vi "Topo & GridSpectr_DriftCorrection_v3.vi"(6 "Internal use":string, 7 "Grid param":T2 {"height (m)" format="%#_6p"; "width (m)" format="%#_6p"; "center Y (m)" format="%#_6p"; "center X (m)" format="%#_6p"}, 8 "Error in (no error)":errorcluster, 9 "Points Y/Index Y":i32, 10 "Points X/Index X":i32, 11 "Method":enum16{"init", "run", "end"}(ring)=enum."end") -> (0 "Error out":errorcluster)   [LabVIEW 2014]
doc: "Example of a measurement VI to be used in the \"Experiments on a Grid\" tool as external VI.\n\nThis example measure the topography and spectroscopy data. The spectroscopy measurements are taken on a subgrid. The data are saved to a sxm and a binary file.\n\n- Nanonis Programming Interface -"
uses:
  <userlib>/Nanonis Prog Interface V5/Nanonis Prog Interface.lvlib
panel:
  in  "Drift Correction 2":T1
  out "Numeric":i32
  out "X drift":i32
  out "Y drift":i32
  out "Queue Steps":i32
  in  "StepsBack":i32
  in  "Channel index (0-23)":u8=14
  in  "File name":string
  in  "STS Current":dbl format="%#_6p"
  in  "Imaging Current":dbl format="%#_6p"
  in  "zdrift \nDuration (s)":dbl
  in  "Correct z drift":bool
  out "Status":string="init"
  in  "Drift correction Pixels":i32=128 caption="Pixels for drift correction"
  out "Y Offset":dbl
  out "X Offset":dbl
  out "Points taken":dbl=1.0
  in  "Drift Correction":i32=128
  in  "Y subgrid spacing":u16=1
  in  "X subgrid spacing":u16=1
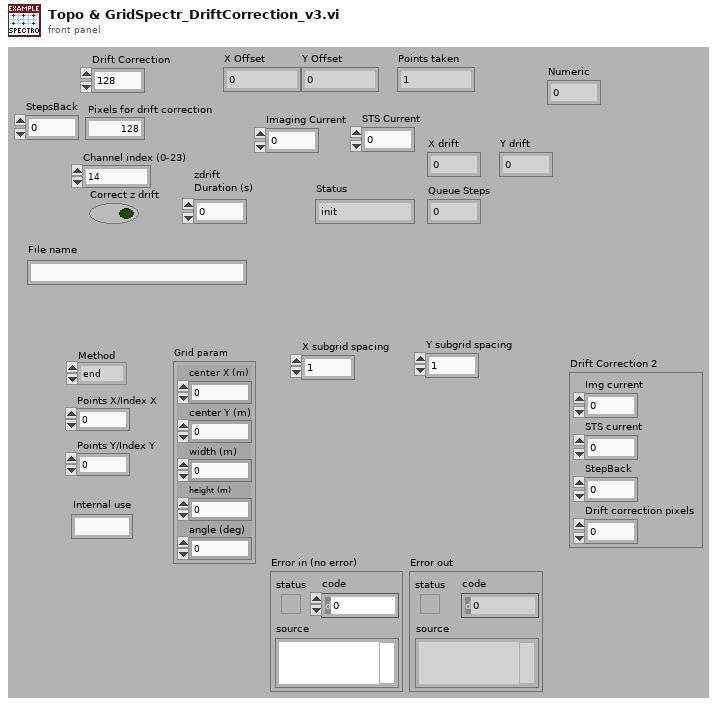
[diagram p1: front panel]
types:
  T1 = cluster{"Img current":dbl, "STS current":dbl, "StepBack":dbl, "Drift correction pixels":dbl}
  T2 = cluster{"center X (m)":sgl, "center Y (m)":sgl, "width (m)":sgl, "height (m)":sgl, "angle (deg)":sgl}
  T3 = cluster{"center X":sgl, "center Y":sgl, "angle":sgl, "width":sgl, "height":sgl, "# pixels":i32, "# lines":i32}
  T4 = cluster{"Name":string, "Calibration":sgl, "Offset":sgl, "Channel index":i32}[]
  T5 = cluster{"up/down":bool, "time/line":sgl, "start time":timestamp, "end time":timestamp}
  T6 = cluster{"Z averaging time (s)":sgl, "Z offset (m)":sgl, "Initial settling time (s)":sgl}
  T7 = cluster{"Max. slew rate (V/s)":sgl, "Settling time (s)":sgl, "Integration time (s)":sgl}
  T8 = cluster{"End settling time (s)":sgl, "Z control time (s)":sgl}
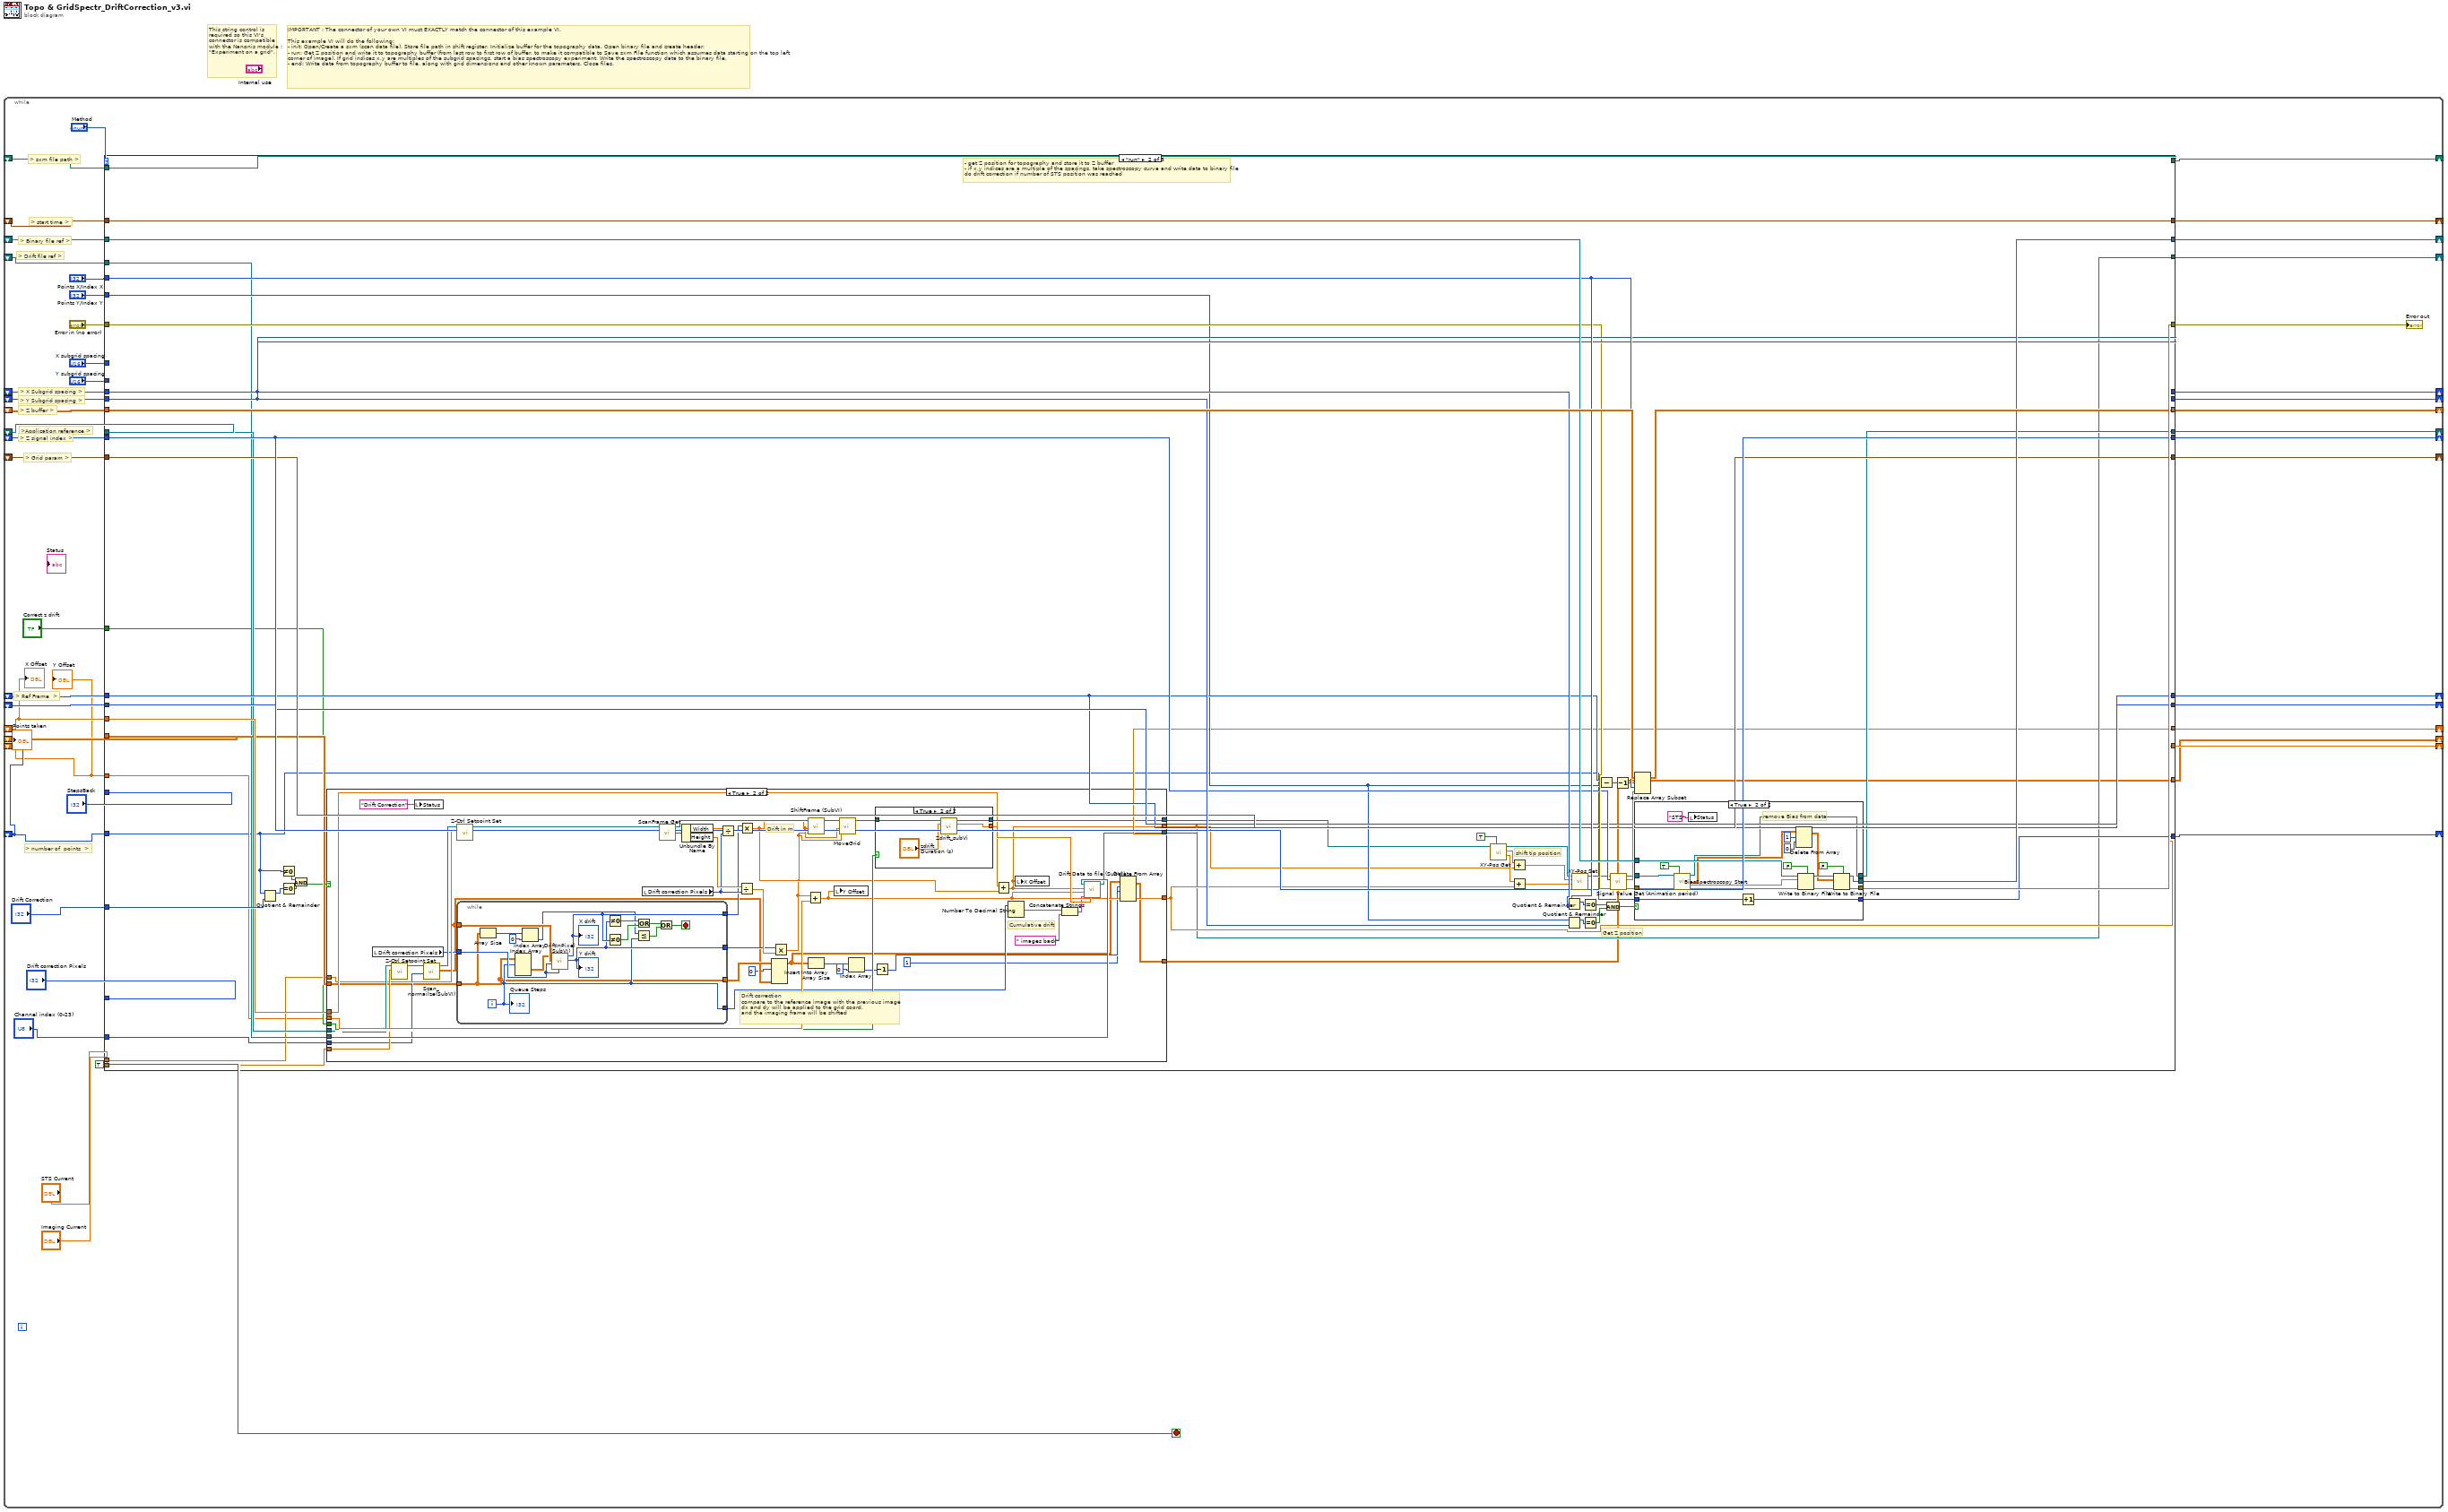
[diagram p0: block diagram]
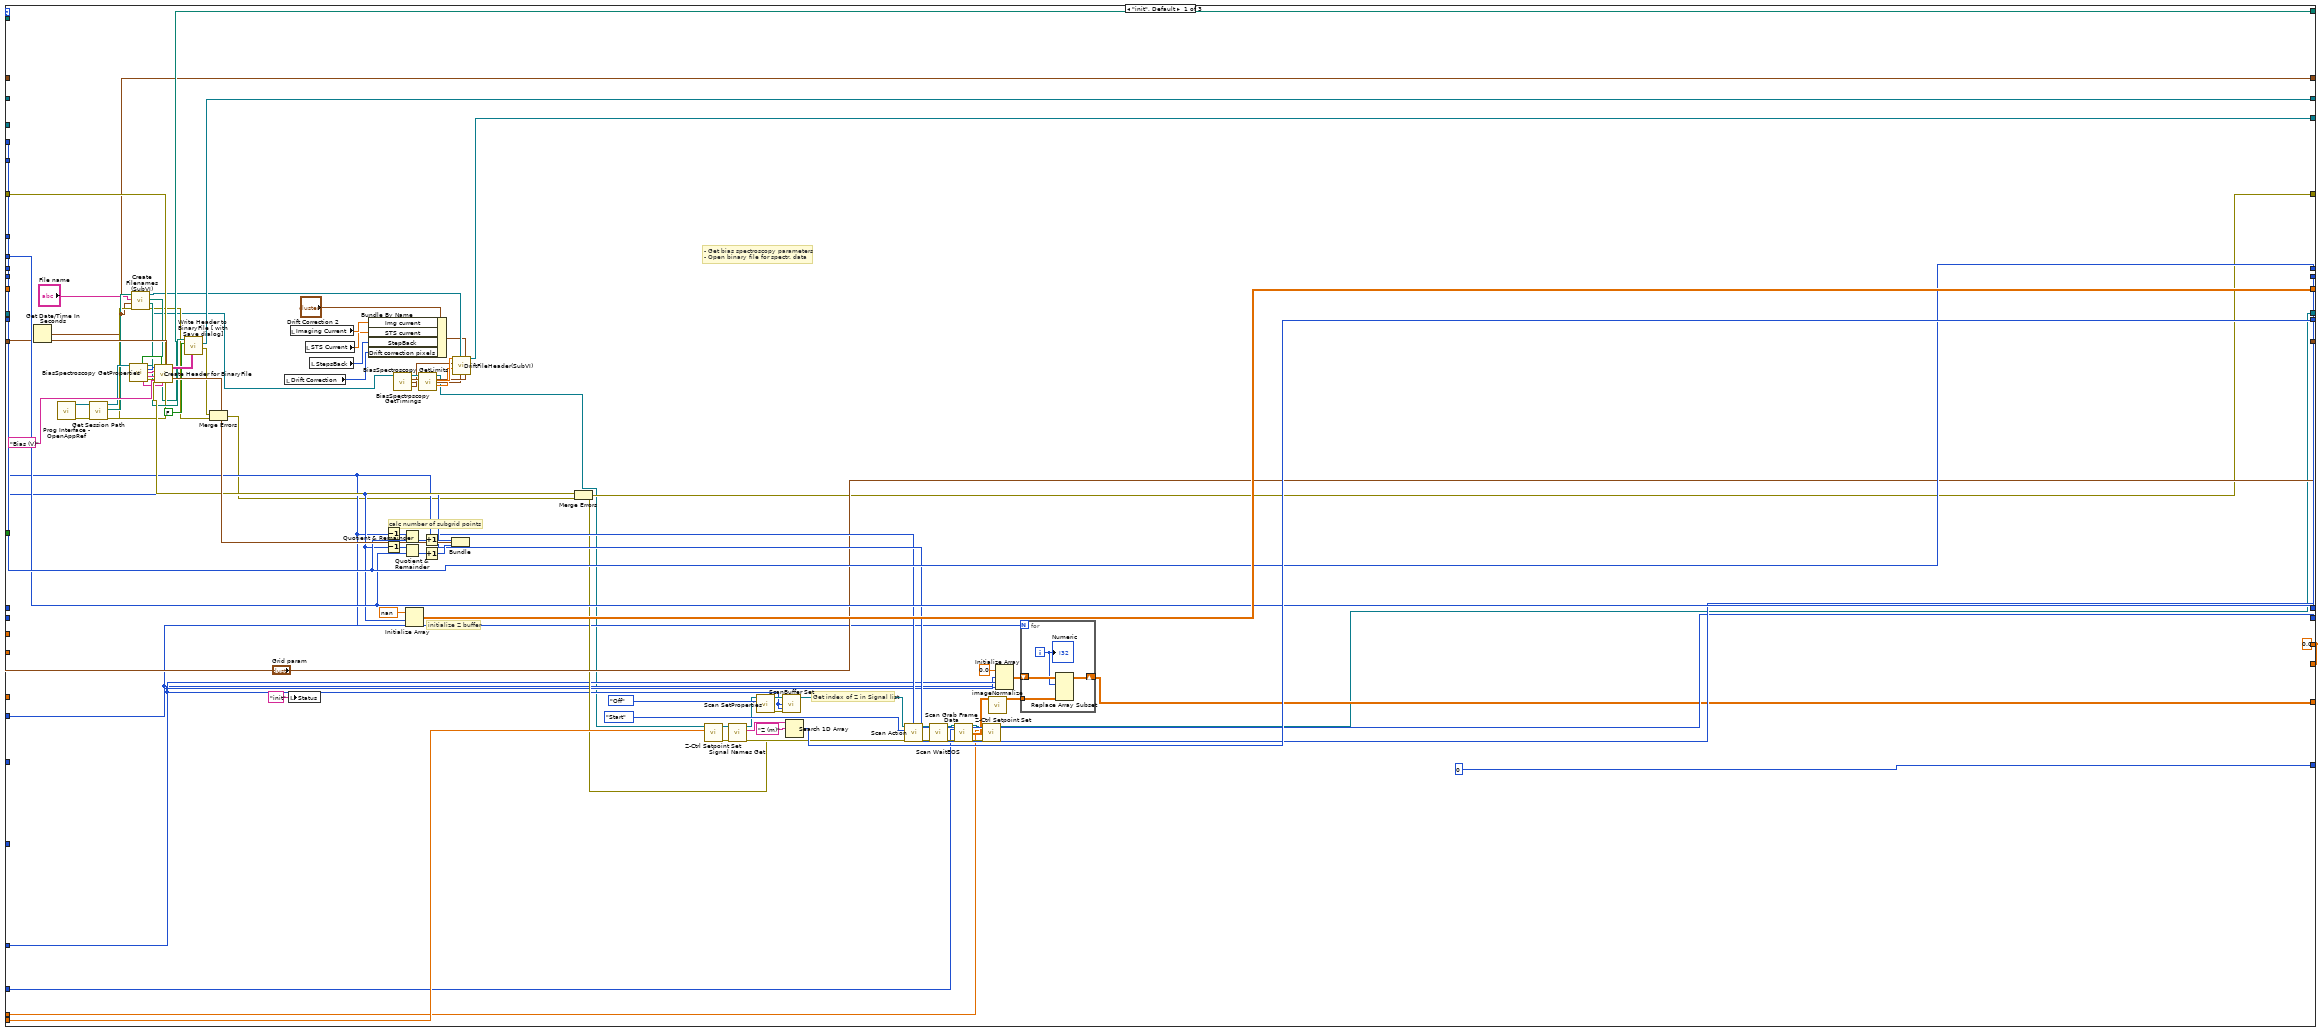
[diagram p2: hidden frame]
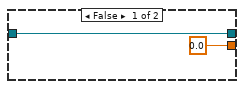
[diagram p4: hidden frame]
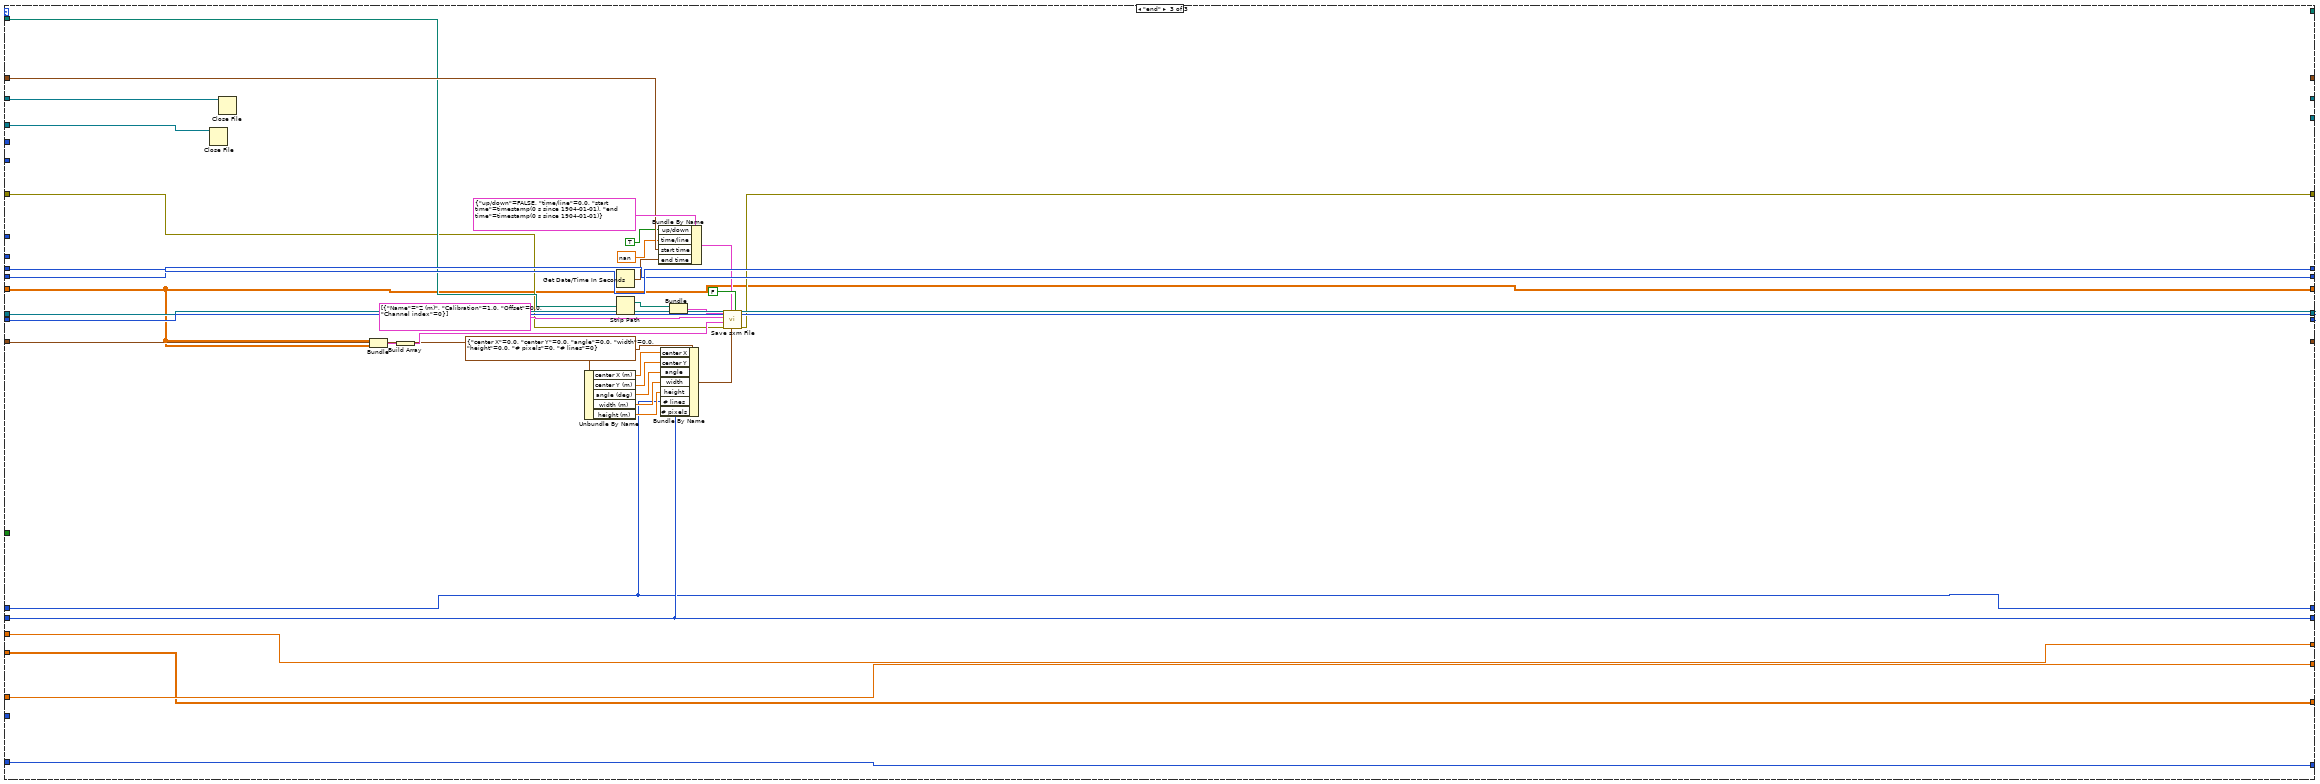
[diagram p6: hidden frame]
diagram:
  # "This string control is required so this VI's connector is compatible with the Nanonis module : \"Experiment on a grid\"."
  # "IMPORTANT : The connector of your own VI must EXACTLY match the connector of this example VI.\n\nThis example VI will do the following:\n- init: Open/Create a sxm (scan data file). Store file path in shift register. Initialize buffer for the topography data. Open binary file and create header.\n- run: Get Z position and write it to topography buffer (from last row to first row of buffer, to make it compatible to Save sxm File function which assumes data starting on the top left corner of image). If grid indices x,y are multiples of the subgrid spacings, start a bias spectroscopy experiment. Write the spectroscopy data to the binary file.\n- end: Write data from topography buffer to file, along with grid dimensions and other known parameters. Close files."
  n1 = while {
    shift-right: [w22] -> _
    shift-left: _ -> [w45]
    shift-right: [w40] -> _
    shift-left: _ -> [w39]
    shift-right: [w37] -> _
    shift-left: _ -> [w38]
    shift-right: [w36] -> _
    shift-left: _ -> [w35]
    shift-right: [w29] -> _
    shift-left: _ -> [w31]
    shift-right: [w30] -> _
    shift-left: _ -> [w32]
    shift-right: [w28] -> _
    shift-left: _ -> [w27]
    shift-right: [w26] -> _
    shift-left: _ -> [w25]
    shift-right: [w24] -> _
    shift-left: _ -> [w23]
    shift-right: [w21] -> _
    shift-left: _ -> [w20]
    shift-right: [w19] -> _
    shift-left: _ -> [w18]
    shift-right: [w17] -> _
    shift-left: _ -> [w10]
    shift-right: [w16] -> _
    shift-left: _ -> [w9]
    shift-right: [w15] -> _
    shift-left: _ -> [w12]
    shift-right: [w14] -> _
    shift-left: _ -> [w11]
    shift-right: [w7] -> _
    shift-left: _ -> [w6]
    stop <- TRUE stop-if-true
    # "> Drift file ref >"
    # "> number of  points  >"
    # "> Ref Frame  >"
    # "> Grid param >"
    # "> start time >"
    # ">Application reference >"
    # "> Y Subgrid spacing >"
    # "> X Subgrid spacing >"
    # "> Z signal index >"
    # "> Binary file ref >"
    # "> Z buffer >"
    # "> sxm file path >"
    n2 = case shown="\"run\"" "Method" {
      tunnel: [w77 w192 _] -> w22
      tunnel: w45 -> [_ w192 w315]
      tunnel: "Error in (no error)" -> [w79 w178 w308]
      tunnel: [w88 w191 w307] -> w43
      tunnel: "Points X/Index X" -> [w109 w186 _]
      tunnel: "Points Y/Index Y" -> [w110 w170 _]
      tunnel: [w133 w189 w296] -> w40
      tunnel: w39 -> [_ w190 w296]
      tunnel: w38 -> [_ w188 w324]
      tunnel: [w125 w187 _] -> w37
      tunnel: [w123 w176 w325] -> w36
      tunnel: w35 -> [_ w176 w325]
      tunnel: "X subgrid spacing" -> [w122 _ _]
      tunnel: "Y subgrid spacing" -> [w121 _ _]
      tunnel: w32 -> [_ w180 w323]
      tunnel: w31 -> [_ w179 w322]
      tunnel: [w122 w180 w323] -> w30
      tunnel: [w121 w179 w322] -> w29
      tunnel: [w50 w162 w321] -> w28
      tunnel: w27 -> [_ w161 w321]
      tunnel: ["Grid param" w173 _] -> w26
      tunnel: w25 -> [_ w173 w306]
      tunnel: [w76 w174 _] -> w24
      tunnel: w23 -> [_ w174 w316]
      tunnel: [w110 w171 w297] -> w21
      tunnel: w20 -> [_ w171 w297]
      tunnel: [w109 w172 w298] -> w19
      tunnel: w18 -> [_ w172 w298]
      tunnel: [w100 w146 w295] -> w17
      tunnel: [w100 w151 w293] -> w16
      tunnel: [w71 w143 w289] -> w15
      tunnel: [0 w167 w294] -> w14
      tunnel: w11 -> [_ w140 w294]
      tunnel: "Drift Correction" -> [_ w165 _]
      tunnel: w12 -> [_ w150 w289]
      tunnel: w10 -> [_ w163 w295]
      tunnel: w9 -> [_ w141 w293]
      tunnel: "Drift correction Pixels" -> [w70 _ _]
      tunnel: [w66 w148 _] -> w7
      tunnel: w6 -> [_ w149 w290]
      tunnel: "Correct z drift" -> [_ w147 _]
      tunnel: "Imaging Current" -> [w89 w145 _]
      tunnel: "STS Current" -> [w84 w144 _]
      tunnel: "Channel index (0-23)" -> [w74 w142 _]
      tunnel: "StepsBack" -> [w69 _ _]
      frame "init", Default {
        w100 = 0.0
        # "- Get bias spectroscopy parameters\n- Open binary file for spectr. data"
        # "initialize Z buffer"
        # "calc number of subgrid points"
        # "Get index of Z in Signal list"
        n3 = Get Date/Time In Seconds() -> (seconds since 1Jan1904=w76:timestamp)
        n4 = call <userlib>:"Prog Interface - OpenAppRef.vi"("Error in (no error)"=w79) -> ("Error out"=w81:errorcluster, "Application reference"=w83:refnum<vi>)  [unwired: 5 in]
        n5 = call <userlib>:"Get Session Path.vi"("error in (no error)"=w81, "Application ref in"=w83) -> ("error out"=w78:errorcluster, "Session path"=w80:path, "Application ref out"=w82:refnum<vi>)  [unwired: 7 in]
        n6 = call <userlib>:"BiasSpectroscopy GetProperties.vi"("Application ref in"=w82) -> ("Backward sweep"=w129:bool, "Application ref out"=w49:refnum<vi>, "Number of points"=w112:i32, "Channels"=w111:string[], "Parameters"=w127:string[], "Fixed parameters"=w114:string[], "Error out"=w126:errorcluster)  [unwired: 6 in, 2 out]
        n7 = call "Create Filenames (SubVI).vi"("error in (no error)"=w78, "seconds since 1Jan1904"=w76, "File name"="File name", "Session path"=w80) -> ("error out"=w51:errorcluster, "binFilePath"=w92:path, "topoFilePath"=w77:path, "Drift File out"=w67:refnum<file>)  [unwired: 4 in]
        n8 = local read "Drift Correction"() -> (w61:i32)
        n9 = local write "Status"("init" ("Status")) -> ()
        n10 = local read "Imaging Current"() -> (w63:dbl)
        n11 = local read "STS Current"() -> (w62:dbl)
        n12 = local read "StepsBack"() -> (w60:i32)
        n13 = Bundle By Name(cluster="Drift Correction 2", "Img current"=w63, "STS current"=w62, "StepBack"=w60, "Drift correction pixels"=w61) -> (w64:T1)
        n14 = Decrement(x=w109) -> (x-1=w120:i32)
        n15 = Decrement(x=w110) -> (x-1=w119:i32)
        n16 = call <userlib>:"BiasSpectroscopy GetTimings.vi"("Application ref in"=w49) -> ("Application ref out"=w59:refnum<vi>, "Initialization"=w56:T6, "Sweep Timing"=w54:T7, "End of Sweep"=w55:T8)  [unwired: 10 in, 1 out]
        n17 = Quotient & Remainder(x=w120, y=w122) -> (floor(x/y)=w118:i32)  [unwired: 1 out]
        n18 = Quotient & Remainder(x=w119, y=w121) -> (floor(x/y)=w117:i32)  [unwired: 1 out]
        n19 = Initialize Array(sgl nan ("element"), w110, w109) -> (w133:sgl[][])
        n20 = call <userlib>:"BiasSpectroscopy GetLimits.vi"("Application ref in"=w59) -> ("End value (V)"=w57:sgl, "Start value (V)"=w58:sgl, "Application ref out"=w48:refnum<vi>)  [unwired: 5 in, 1 out]
        n21 = Increment(x=w118) -> (x+1=w116:i32)
        n22 = Increment(x=w117) -> (x+1=w115:i32)
        n23 = Bundle(w116, w115) -> (w128:cluster{i32, i32})  [unwired: 1 in]
        n24 = call <userlib>:"Create Header for BinaryFile.vi"("Grid points"=w128, "Grid param"="Grid param", "Fixed parameters"=w114, "Backward sweep"=w129, "Sweep signal"="Bias (V)" ("Sweep Signal"), "Parameters"=w127, "Channels"=w111, "Points per sweep"=w112) -> ("Header (fixed attributes)"=w131:string[][])  [unwired: 3 in]
        n25 = call <userlib>:"Write Header to BinaryFile [ with Save dialog].vi"("Fixed Attributes"=w131, "Show Dialog? (T)"=FALSE, "Filename"=w92) -> ("Error out"=w52:errorcluster, "File ref"=w125:refnum<file>)  [unwired: 5 in, 2 out]
        n26 = Merge Errors(w52, w51) -> (w53:errorcluster)
        n27 = call "DriftFileHeader(SubVI).vi"("Initialization"=w56, "Drift Correction"=w64, "Sweep Timing"=w54, "Byte Stream File in"=w67, "End value (V)"=w57, "End of Sweep"=w55, "Start value (V)"=w58) -> ("Byte Stream File out"=w66:refnum<file>)  [unwired: 4 in]
        n28 = Merge Errors(w126, w53) -> (w88:errorcluster)
        n29 = call <userlib>:"Z-Ctrl Setpoint Set.vi"("error in (no error)"=w88, "Z Controller setpoint"=w89, "Application ref in"=w48) -> ("error out"=w87:errorcluster, "Application ref out"=w90:refnum<vi>)  [unwired: 7 in]
        n30 = call <userlib>:"Signal Names Get.vi"("error in (no error)"=w87, "Application ref in"=w90) -> ("error out"=w101:errorcluster, "Signals Names"=w113:string[], "Application ref out"=w96:refnum<vi>)  [unwired: 5 in]
        n31 = call <userlib>:"Scan SetProperties.vi"("Application ref in"=w96, "Continuous scan"=enum16{"No change", "On", "Off"}."Off") -> ("Application ref out"=w98:refnum<vi>, "Error out"=w97:errorcluster)  [unwired: 12 in]
        n32 = call <userlib>:"ScanBuffer Set.vi"("Application ref in"=w98, "Pixels"=w70, "Lines"=w70, "error in (no error)"=w97) -> ("Application ref out"=w95:refnum<vi>)  [unwired: 10 in, 1 out]
        n33 = Search 1D Array(1D array=w113, element="Z (m)") -> (index of element=w123:i32)  [unwired: 1 in]
        n34 = call <userlib>:"Scan Action.vi"("error in (no error)"=w101, "Scan action (Start)"=enum16{"Start", "Stop", "Pause", "Resume"}."Start", "Application ref in"=w95) -> ("error out"=w107:errorcluster, "Application ref out"=w106:refnum<vi>)  [unwired: 6 in]
        n35 = call <userlib>:"Scan WaitEOS.vi"("error in (no error)"=w107, "Application ref in"=w106) -> ("error out"=w104:errorcluster, "Application ref out"=w105:refnum<vi>)  [unwired: 5 in, 2 out]
        n36 = call <userlib>:"Scan Grab Frame Data.vi"("Application ref in"=w105, "Channel index (0-23)"=w74, "error in (no error)"=w104) -> ("Application ref out"=w86:refnum<vi>, "Scan frame data"=w91:sgl[][], "error out"=w85:errorcluster)  [unwired: 8 in, 2 out]
        n37 = call <userlib>:"Z-Ctrl Setpoint Set.vi"("error in (no error)"=w85, "Z Controller setpoint"=w84, "Application ref in"=w86) -> ("Application ref out"=w50:refnum<vi>)  [unwired: 7 in, 1 out]
        n38 = call "imageNormalize.vi"("Data"=w91) -> ("Array"=w68:dbl[][])  [unwired: 10 in]
        n39 = Initialize Array(0.0 ("element"), w69, w70, w70) -> (w72:dbl[][][])
        n40 = for {
          N: w69 -> [_]
          tunnel: w68 -> [w136]
          shift-right: [w135] -> w71
          shift-left: w72 -> [w137]
          i -> [w134]
          n41 = Replace Array Subset(array=w137, new element=w136, index (dim 0)=w134) -> (w135:dbl[][][])  [unwired: 2 in]
          "Numeric" <- w134
        }
      }
      frame "run" {
        # "shift tip position"
        # "Get Z position"
        # "- get Z position for topography and store it to Z buffer\n- if x,y indices are a multiple of the spacings, take spectroscopy curve and write data to binary file\ndo drift correction if number of STS position was reached"
        n42 = Quotient & Remainder(x=w140, y=w165) -> (x-y*floor(x/y)=w166:i32)  [unwired: 1 out]
        n43 = Not Equal To 0?(x=w140) -> (x != 0?=w138:bool)
        n44 = Equal To 0?(x=w166) -> (x = 0?=w164:bool)
        n45 = And(x=w138, y=w164) -> (x .and. y?=w139:bool)
        n46 = case shown="True" w139 {
          tunnel: w161 -> [w197 w228]
          tunnel: [w197 w234] -> w160
          tunnel: w150 -> [w194 w216]
          tunnel: [w196 w230] -> w146
          tunnel: [w195 w229] -> w151
          tunnel: w163 -> [w196 w232]
          tunnel: w141 -> [w195 w233]
          tunnel: [w194 w208] -> w143
          tunnel: w149 -> [w193 w237]
          tunnel: [w193 w236] -> w148
          tunnel: w147 -> [_ w231]
          tunnel: w145 -> [_ w227]
          tunnel: w144 -> [_ w225]
          tunnel: w142 -> [_ w220]
          frame False {
          }
          frame True {
            # "Cumulative drift"
            # "Drift in m"
            # "Drift correction \ncompare to the reference image with the previous image \ndx and dy will be applied to the grid coord, \nand the imaging frame will be shifted"
            n47 = local read "Drift correction Pixels"() -> (w219:i32)
            n48 = call <userlib>:"Z-Ctrl Setpoint Set.vi"("Z Controller setpoint"=w227, "Application ref in"=w228) -> ("Application ref out"=w224:refnum<vi>)  [unwired: 8 in, 1 out]
            n49 = local write "Status"("Drift Correction" ("Status")) -> ()
            n50 = call "Scan_normailze(SubVI).vi"("Channel index (0-23)"=w220, "Application in"=w224) -> ("Array"=w210:dbl[][], "Application out"=w226:refnum<vi>)  [unwired: 7 in, 1 out]
            n51 = call <userlib>:"Z-Ctrl Setpoint Set.vi"("Z Controller setpoint"=w225, "Application ref in"=w226) -> ("Application ref out"=w222:refnum<vi>)  [unwired: 8 in, 1 out]
            n52 = while {
              tunnel: w219 -> [w256]
              tunnel: w210 -> [w255]
              tunnel: w216 -> [w245]
              tunnel: [w254] -> w218
              tunnel: [w253] -> w217
              tunnel: [w249] -> w215
              tunnel: [w245] -> w211
              i -> [w249]
              stop <- w251 stop-if-true
              n53 = Array Size(array=w245) -> (size(s)=w248:i32[])
              n54 = Index Array(array=w245, index (dim 0)=w249) -> (element=w244:dbl[][])  [unwired: 2 in]
              n55 = Index Array(array=w248, index=0) -> (element=w246:i32)
              n56 = call "DriftInPixel (SubVI).vi"(6:w256, 9:w256, "New image"=w255, "Ref image"=w244) -> ("Y drift"=w253:i32, "X drift"=w254:i32)  [unwired: 5 in, 1 out]
              "Y drift" <- w253
              "X drift" <- w254
              n57 = Not Equal To 0?(x=w253) -> (x != 0?=w258:bool)
              n58 = Not Equal To 0?(x=w254) -> (x != 0?=w257:bool)
              n59 = Or(x=w258, y=w257) -> (x .or. y?=w252:bool)
              n60 = Less Or Equal?(x=w246, y=w249) -> (x <= y?=w250:bool)
              n61 = Or(x=w252, y=w250) -> (x .or. y?=w251:bool)
              "Queue Steps" <- w249
            }
            n62 = local read "Drift correction Pixels"() -> (w221:i32)
            n63 = call <userlib>:"ScanFrame Get.vi"("Application ref in"=w222) -> ("Application ref out"=w223:refnum<vi>, "Size (m)"=w242:cluster{"Width":sgl, "Height":sgl})  [unwired: 10 in, 3 out]
            n64 = Unbundle By Name(w242) -> ("Width"=w241:sgl, "Height"=w243:sgl)
            n65 = Divide(x=w241, y=w221) -> (x/y=w240:sgl)
            n66 = Divide(x=w243, y=w221) -> (x/y=w239:sgl)
            n67 = Multiply(x=w218, y=w240) -> (x*y=w199:sgl)
            n68 = Insert Into Array(array=w211, index (dim 0)=0 ("index (page)"), new element=w210) -> (w207:dbl[][][])  [unwired: 2 in]
            n69 = Multiply(x=w217, y=w239) -> (x*y=w198:sgl)
            n70 = Add(x=w198, y=w233) -> (x+y=w229:dbl)
            n71 = call "ShiftFrame (SubVI).vi"("Y shift"=w198, "X shift"=w199, "Application in"=w223) -> ("Application out"=w201:refnum<vi>)  [unwired: 8 in]
            n72 = Array Size(array=w207) -> (size(s)=w206:i32[])
            n73 = local write "Y Offset"(w229) -> ()
            n74 = call "MoveGrid.vi"("y"=w198, "x"=w199, "Application ref in"=w201) -> ("Application ref out"=w200:refnum<vi>)  [unwired: 7 in, 1 out]
            n75 = Index Array(array=w206, index=0) -> (element=w204:i32)
            n76 = Decrement(x=w204) -> (x-1=w203:i32)
            n77 = case shown="True" w231 {
              tunnel: [0.0 ("z drift") w264] -> w235
              tunnel: w200 -> [w259 w263]
              tunnel: [w259 w262] -> w234
              frame False {
              }
              frame True {
                n78 = call "Zdrift_subVi.vi"("Duration"="zdrift \nDuration (s)", "Application in"=w263) -> ("z drift"=w264:dbl, "Application out"=w262:refnum<vi>)  [unwired: 7 in, 1 out]
              }
            }
            n79 = Add(x=w232, y=w199) -> (x+y=w230:dbl)
            n80 = Number To Decimal String(number=w215) -> (decimal integer string=w214:string)  [unwired: 1 in]
            n81 = local write "X Offset"(w230) -> ()
            n82 = Concatenate Strings(w214, " images back" ("string")) -> (w213:string)
            n83 = call "Drift Data to file (SubVI).vi"("z drift"=w235, "Comment"=w213, "y Drift"=w229, "X drift"=w230, "Byte Stream File in"=w237) -> ("Byte Stream File out"=w236:refnum<file>)  [unwired: 6 in]
            n84 = Delete From Array(array=w207, length=1, index (dim 0)=w203) -> (array with subset deleted=w208:dbl[][][])  [unwired: 2 in, 1 out]
          }
        }
        n85 = call <userlib>:"XY-Pos Get.vi"("Wait for newest data (F=False)"=TRUE, "Application ref in"=w160) -> ("Y (m)"=w155:sgl, "X (m)"=w156:sgl, "Application ref out"=w157:refnum<vi>)  [unwired: 5 in, 1 out]
        n86 = Add(x=w156, y=w146) -> (x+y=w154:dbl)
        n87 = Add(x=w155, y=w151) -> (x+y=w153:dbl)
        n88 = Quotient & Remainder(x=w186, y=w180) -> (x-y*floor(x/y)=w185:i32)  [unwired: 1 out]
        n89 = Quotient & Remainder(x=w170, y=w179) -> (x-y*floor(x/y)=w184:i32)  [unwired: 1 out]
        n90 = call <userlib>:"XY-Pos Set.vi"("Y (m)"=w153, "X (m)"=w154, "Application ref in"=w157) -> ("Application ref out"=w158:refnum<vi>)  [unwired: 5 in, 1 out]
        n91 = Equal To 0?(x=w185) -> (x = 0?=w183:bool)
        n92 = Equal To 0?(x=w184) -> (x = 0?=w182:bool)
        n93 = Subtract(x=w171, y=w170) -> (x-y=w169:i32)
        n94 = And(x=w183, y=w182) -> (x .and. y?=w181:bool)
        n95 = call <userlib>:"Signal Value Get (Animation period).vi"("error in (no error)"=w178, "Signal index (0-47)"=w176, "Application ref in"=w158) -> ("error out"=w177:errorcluster, "Signal value"=w175:sgl, "Application ref out"=w159:refnum<vi>)  [unwired: 5 in]
        n96 = Decrement(x=w169) -> (x-1=w168:i32)
        n97 = Replace Array Subset(array=w190, new element=w175, index (row)=w168, index (col)=w186) -> (w189:sgl[][])
        n98 = case shown="True" w181 {
          tunnel: [w267 w272] -> w191
          tunnel: w188 -> [w268 w288]
          tunnel: [w268 w286] -> w187
          tunnel: w177 -> [w267 w285]
          tunnel: w159 -> [w266 w277]
          tunnel: [w266 w276] -> w162
          tunnel: [w265 w270] -> w167
          tunnel: w140 -> [w265 w271]
          frame False {
            # "Point indices aren't multiple of subgrid spacing\n=> no spectroscopy at this point"
          }
          frame True {
            # "remove Bias from data"
            n99 = call <userlib>:"BiasSpectroscopy Start.vi"("Application ref in"=w277, "Get data (F)"=TRUE ("Get Data (F)"), "Error in (no error)"=w285) -> ("Application ref out"=w276:refnum<vi>, "Data"=w284:sgl[][], "Parameters"=w283:sgl[], "Error out"=w274:errorcluster)  [unwired: 8 in, 1 out]
            n100 = local write "Status"("STS" ("Status")) -> ()
            n101 = Increment(x=w271) -> (x+1=w270:i32)
            n102 = Delete From Array(array=w284, length=1, index (row)=0 ("index")) -> (array with subset deleted=w282:sgl[][])  [unwired: 1 in, 1 out]
            n103 = Write to Binary File(file (use dialog)=w288, data=w283, error in=w274, 5:FALSE ("prepend array or string size? (T)")) -> (refnum out=w287:refnum<file>, error out=w273:errorcluster)  [unwired: 2 in, 1 out]
            n104 = Write to Binary File(file (use dialog)=w287, data=w282, error in=w273, 5:FALSE ("prepend array or string size? (T)")) -> (refnum out=w286:refnum<file>, error out=w272:errorcluster)  [unwired: 2 in, 1 out]
          }
        }
      }
      frame "end" {
        n105 = Close File(refnum=w290) -> ()  [unwired: 1 in, 2 out]
        n106 = Close File(refnum=w324) -> ()  [unwired: 1 in, 2 out]
        n107 = Bundle(w296, w296) -> (w320:cluster{sgl[][], sgl[][]})  [unwired: 1 in]
        n108 = Build Array(w320) -> (w319:cluster{sgl[][], sgl[][]}[])
        n109 = Unbundle By Name(w306) -> ("center X (m)"=w304:sgl, "center Y (m)"=w303:sgl, "angle (deg)"=w302:sgl, "width (m)"=w301:sgl, "height (m)"=w300:sgl)
        n110 = Get Date/Time In Seconds() -> (seconds since 1Jan1904=w292:timestamp)
        n111 = Strip Path(path=w315) -> (stripped path=w311:path, name=w310:string)
        n112 = Bundle By Name(cluster=T5 {"up/down"=FALSE, "time/line"=0.0, "start time"=timestamp(0 s since 1904-01-01), "end time"=timestamp(0 s since 1904-01-01)} ("Scan param"), "up/down"=TRUE, "time/line"=sgl nan ("input 7"), "start time"=w316, "end time"=w292) -> (w314:T5)
        n113 = Bundle By Name(cluster=T3 {"center X"=0.0, "center Y"=0.0, "angle"=0.0, "width"=0.0, "height"=0.0, "# pixels"=0, "# lines"=0} ("Scanfield"), "center X"=w304, "center Y"=w303, "angle"=w302, "width"=w301, "height"=w300, "# lines"=w297, "# pixels"=w298) -> (w299:T3)
        n114 = Bundle("stripped path"=w311, "name"=w310) -> (w309:cluster{"stripped path":path, "name":string})  [unwired: 1 in]
        n115 = call <userlib>:"Save sxm File.vi"("Auto file naming? (T)"=FALSE, "Scanfield"=w299, "Scan param"=w314, "error in (no error)"=w308, "Channels data"=w319, "Channels config"=T4 [{"Name"="Z (m)", "Calibration"=1.0, "Offset"=0.0, "Channel index"=0}], "Filename control"=w309) -> ("error out"=w307:errorcluster)  [unwired: 2 in, 2 out]
      }
    }
    "Error out" <- w43
    "Points taken" <- w11
    "X Offset" <- w10
    "Y Offset" <- w9
  }
